vi "Calling Python Script.vi"(3 "error in (no error)":errorcluster, 5 "Path":path=path "C:/Users/stefan/Documents/GitHub/TVAC/head/Labview2017/TVAC_GUI/TestScripts/graphTest.json") -> (0 "error out":errorcluster, 2 "graphCluster":T1)   [LabVIEW 2017]
panel:
  in  "Path to Python.exe":path=path "C:/ProgramData/Anaconda3/python.exe"
  out "Raw Python String Output":string
  out "Standard Error":string
  out "Return Code":i32
  # "1. Inputs - Set before running VI"
  # "2. Outputs"
  # "3. Errors - Both Standard and LabVIEW"
  # "A + B ="
  # "This VI sends inputs to a simple Python script, and returns its output.\n\nSee block diagram for code and comments"
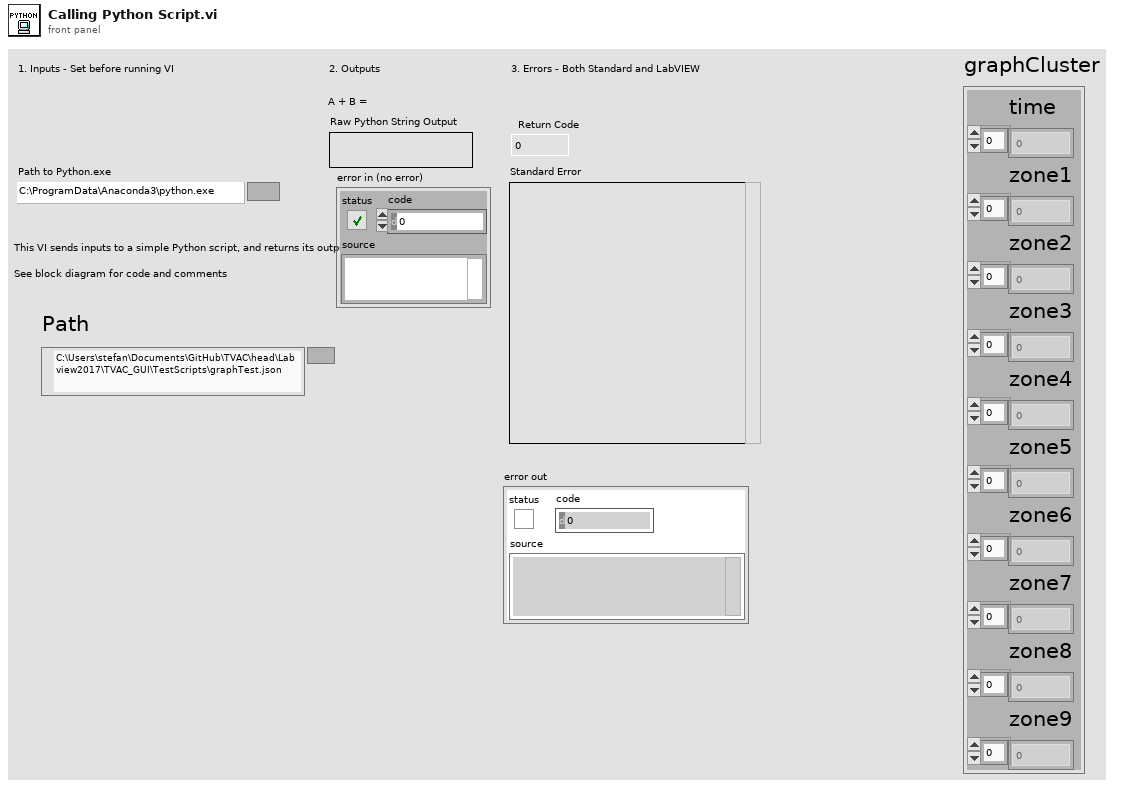
[diagram p1: front panel]
types:
  T1 = cluster{"time":dbl[], "zone1":dbl[], "zone2":dbl[], "zone3":dbl[], "zone4":dbl[], "zone5":dbl[], "zone6":dbl[], "zone7":dbl[], "zone8":dbl[], "zone9":dbl[]}
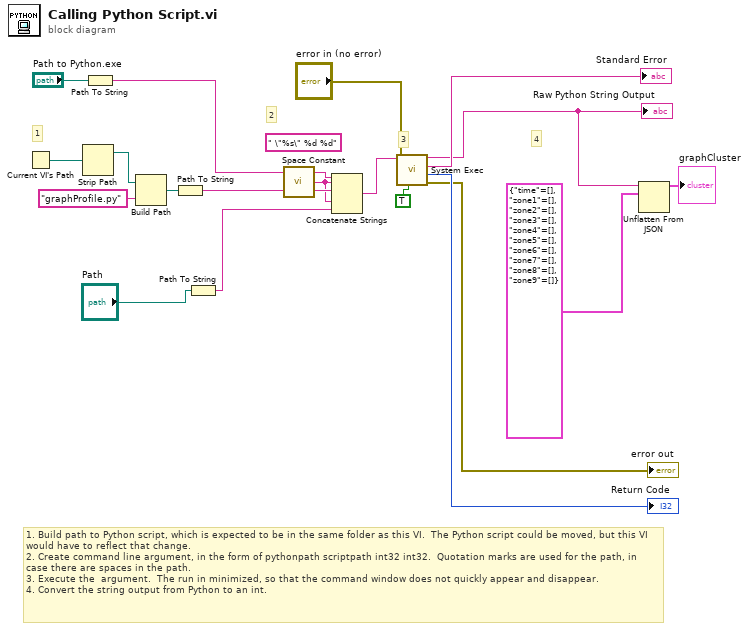
[diagram p0: block diagram]
diagram:
  (unwired) " \"%s\" %d %d" ("format string")
  # "1. Build path to Python script, which is expected to be in the same folder as this VI.  The Python script could be moved, but this VI would have to reflect that change.\n2. Create command line argument, in the form of pythonpath scriptpath int32 int32.  Quotation marks are used for the path, in case there are spaces in the path.\n3. Execute the  argument.  The run in minimized, so that the command window does not quickly appear and disappear.\n4. Convert the string output from Python to an int."
  # "4"
  # "3"
  # "2"
  # "1"
  n1 = Current VI's Path() -> (path=w14:path)
  n2 = Strip Path(path=w14) -> (stripped path=w12:path)  [unwired: 1 out]
  n3 = Path To String(path="Path to Python.exe") -> (string=w8:string)
  n4 = Build Path(base path=w12, name or relative path="graphProfile.py" ("Path to Function")) -> (appended path=w15:path)
  n5 = Path To String(path=w15) -> (string=w9:string)
  n6 = Path To String(path="Path") -> (string=w5:string)
  n7 = call <vilib>:"Space Constant.vi"() -> ("String"=w7:string)
  n8 = Concatenate Strings(w8, w7, w9, w7, w5) -> (w10:string)
  n9 = call <vilib>:"System Exec.vi"("run minimized? (F)"=TRUE, "error in (no error)"="error in (no error)", "command line"=w10) -> ("error out"=→"error out":errorcluster, "return code"=→"Return Code":i32, "standard error"=→"Standard Error":string, "standard output"=w3:string)  [unwired: 5 in]
  "Raw Python String Output" <- w3
  n10 = Unflatten From JSON(JSON string=w3, type and defaults=T1 {"time"=[], "zone1"=[], "zone2"=[], "zone3"=[], "zone4"=[], "zone5"=[], "zone6"=[], "zone7"=[], "zone8"=[], "zone9"=[]}) -> (value=→"graphCluster":T1)  [unwired: 5 in, 1 out]
